vi "Equalize Channel (FIR).vi"(0 "input data":cdb[](array[numeric])=array[8192 elements], 5 "FIR coeff":cdb[](array[numeric])=array[8192 elements]) -> (3 "processing time":dbl format="%#_6p", 4 "output data":cdb[](array[numeric]))   [LabVIEW 2019]
uses:
  f2039055-3924-407a-8a5b-c092533b0b2c.vi
  5ecdb60a-3ed6-428b-acf7-caf6d22cb021.vi
  <vilib>/Utility/High Resolution Relative Seconds.vi
  <vilib>/Utility/error.llb/Clear Errors.vi
  <vilib>/Analysis/3filter.llb/FIR Filter (DBL).vi
  <vilib>/Analysis/NI_AALBase.lvlib
  5bce466e-7373-45d0-abac-f28a3138f870.vi
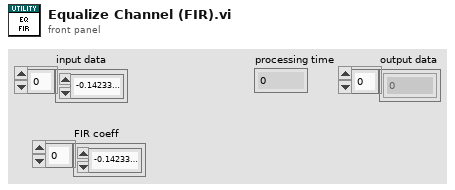
[diagram p1: front panel]
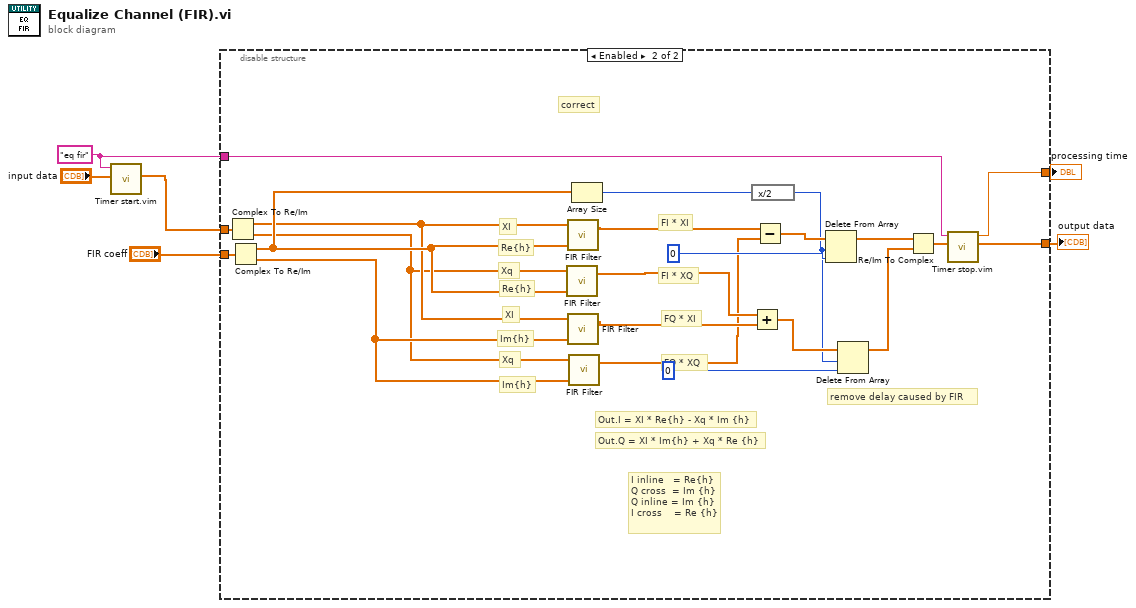
[diagram p0: block diagram]
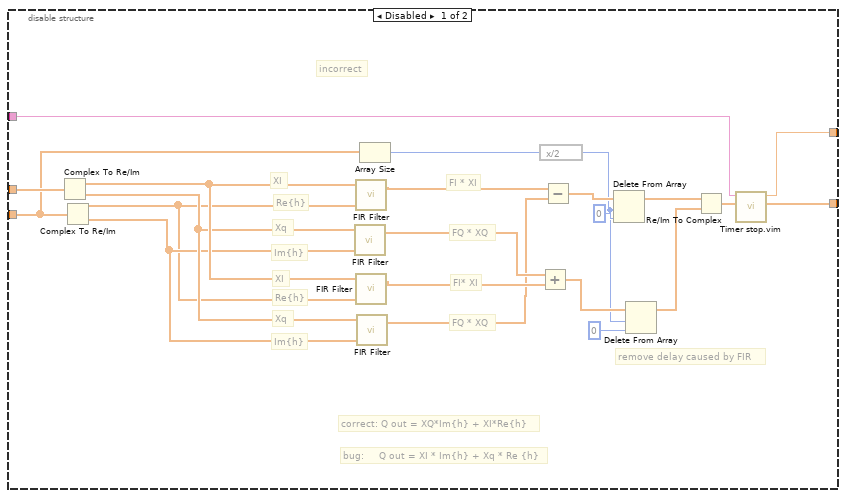
[diagram p2: hidden frame]
diagram:
  w2 = "eq fir" ("timer name (t1)")
  n1 = call "Timer start.vim"("dataflow in"="input data", "timer name (t1)"=w2) -> ("dataflow out"=w4:cdb[])  [unwired: 9 in]
  n2 = disable-structure shown="Enabled" {
    disable-tunnel: "FIR coeff" -> [w9 w34]
    disable-tunnel: w4 -> [w14 w33]
    disable-tunnel: [w12 w31] -> w3
    disable-tunnel: w2 -> [w11 w30]
    disable-tunnel: [w10 w29] -> w1
    frame Disabled {
      # "bug:     Q out = XI * Im{h} + Xq * Re {h}"
      # "correct: Q out = XQ*Im{h} + XI*Re{h}"
      # "Im{h}"
      # "Im{h}"
      # "Re{h}"
      # "Re{h}"
      # "Xq"
      # "Xq"
      # "XI"
      # "XI"
      # "incorrect"
      # "remove delay caused by FIR"
      # "FQ * XQ"
      # "FQ * XQ"
      # "FI* XI"
      # "FI * XI"
      n3 = Complex To Re/Im(x + iy=w14) -> (x=w19:dbl[], y=w17:dbl[])
      n4 = Complex To Re/Im(x + iy=w9) -> (x=w7:dbl[], y=w8:dbl[])
      n5 = call-poly <vilib>:"FIR Filter.vi"("FIR Coefficients"=w8, "X"=w17) -> ("Filtered X"=w21:dbl[])  [unwired: 2 in, 1 out]
      n6 = call-poly <vilib>:"FIR Filter.vi"("FIR Coefficients"=w7, "X"=w19) -> ("Filtered X"=w22:dbl[])  [unwired: 2 in, 1 out]
      n7 = call-poly <vilib>:"FIR Filter.vi"("FIR Coefficients"=w7, "X"=w19) -> ("Filtered X"=w20:dbl[])  [unwired: 2 in, 1 out]
      n8 = call-poly <vilib>:"FIR Filter.vi"("FIR Coefficients"=w8, "X"=w17) -> ("Filtered X"=w18:dbl[])  [unwired: 2 in, 1 out]
      n9 = Array Size(array=w9) -> (size(s)=w23:i32)
      n10 = expression code="x/2"(w23) -> (w24:i32)
      n11 = Add(x=w21, y=w20) -> (x+y=w27:dbl[])
      n12 = Subtract(x=w22, y=w18) -> (x-y=w28:dbl[])
      n13 = Delete From Array(array=w28, length=w24, index=0) -> (array with subset deleted=w16:dbl[])  [unwired: 1 out]
      n14 = Delete From Array(array=w27, length=w24, index=0) -> (array with subset deleted=w15:dbl[])  [unwired: 1 out]
      n15 = Re/Im To Complex(1:w15, 2:w16) -> (0:w13:cdb[])
      n16 = call "Timer stop.vim"("dataflow in"=w13, "timer name (t1)"=w11) -> ("dataflow out"=w12:cdb[], "final time"=w10:dbl)  [unwired: 8 in]
    }
    frame Enabled {
      # "I inline   = Re{h} \nQ cross  = Im {h}\nQ inline = Im {h}\nI cross    = Re {h}"
      # "Out.Q = XI * Im{h} + Xq * Re {h}"
      # "Out.I = XI * Re{h} - Xq * Im {h}"
      # "Xq"
      # "XI"
      # "Im{h}"
      # "Im{h}"
      # "Re{h}"
      # "Xq"
      # "Re{h}"
      # "XI"
      # "correct"
      # "remove delay caused by FIR"
      # "FQ * XQ"
      # "FQ * XI"
      # "FI * XQ"
      # "FI * XI"
      n17 = Complex To Re/Im(x + iy=w33) -> (x=w39:dbl[], y=w37:dbl[])
      n18 = Complex To Re/Im(x + iy=w34) -> (x=w44:dbl[], y=w40:dbl[])
      n19 = call-poly <vilib>:"FIR Filter.vi"("FIR Coefficients"=w44, "X"=w37) -> ("Filtered X"=w42:dbl[])  [unwired: 2 in, 1 out]
      n20 = call-poly <vilib>:"FIR Filter.vi"("FIR Coefficients"=w44, "X"=w39) -> ("Filtered X"=w43:dbl[])  [unwired: 2 in, 1 out]
      n21 = call-poly <vilib>:"FIR Filter.vi"("FIR Coefficients"=w40, "X"=w39) -> ("Filtered X"=w41:dbl[])  [unwired: 2 in, 1 out]
      n22 = call-poly <vilib>:"FIR Filter.vi"("FIR Coefficients"=w40, "X"=w37) -> ("Filtered X"=w38:dbl[])  [unwired: 2 in, 1 out]
      n23 = Array Size(array=w44) -> (size(s)=w45:i32)
      n24 = expression code="x/2"(w45) -> (w46:i32)
      n25 = Add(x=w42, y=w41) -> (x+y=w49:dbl[])
      n26 = Subtract(x=w43, y=w38) -> (x-y=w50:dbl[])
      n27 = Delete From Array(array=w50, length=w46, index=0) -> (array with subset deleted=w36:dbl[])  [unwired: 1 out]
      n28 = Delete From Array(array=w49, length=w46, index=0) -> (array with subset deleted=w35:dbl[])  [unwired: 1 out]
      n29 = Re/Im To Complex(1:w35, 2:w36) -> (0:w32:cdb[])
      n30 = call "Timer stop.vim"("dataflow in"=w32, "timer name (t1)"=w30) -> ("dataflow out"=w31:cdb[], "final time"=w29:dbl)  [unwired: 8 in]
    }
  }
  "output data" <- w3
  "processing time" <- w1
